vi "Throw Invalid Hierarchy.vi"(8 "error in (no error)":errorcluster) -> (0 "error out":errorcluster)   [LabVIEW 2020, in "ExecAnchor.lvclass"]
uses:
  ExecAnchor.lvclass
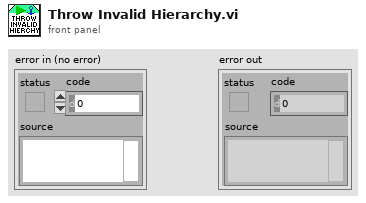
[diagram p1: front panel]
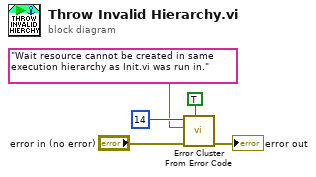
[diagram p0: block diagram]
diagram:
  n1 = call <vilib>:"Error Cluster From Error Code.vi"("show call chain? (False)"=TRUE, "error in (no error)"="error in (no error)", "error message (\"\")"="Wait resource cannot be created in same execution hierarchy as Init.vi was run in." ("error message (\"\")"), "error code (0)"=14) -> ("error out"=→"error out":errorcluster)  [unwired: 5 in]
